vi "Move DC_X_Power.vi"   [LabVIEW 2010, in "4134Outputs.lvlib"]
uses:
  4134Outputs.lvlib
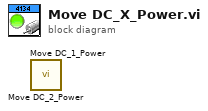
[diagram p0: block diagram]
diagram:
  n1 = call "Move DC_2_Power.vi"() -> ()  [unwired: 10 in, 1 out]
  n2 = call "Move DC_1_Power.vi"() -> ()  [unwired: 10 in, 1 out]
